vi "dfd_Lattice Level Down.vi"(0 "Bm(z)":dbl[](array[numeric]) format="%.2f") -> (1 "Bm-1(z)":dbl[](array[numeric]) format="%.2f", 2 "km":dbl format="%.2f", 3 "fail?":bool)   [LabVIEW 2017, in "NI_DigFilterLicensed.lvlib"]
uses:
  <vilib>/addons/Digital Filter Design/NI_DigFilterLicensed.lvlib
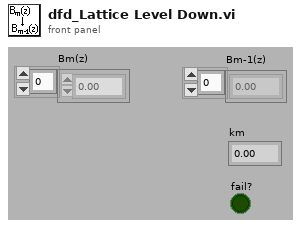
[diagram p1: front panel]
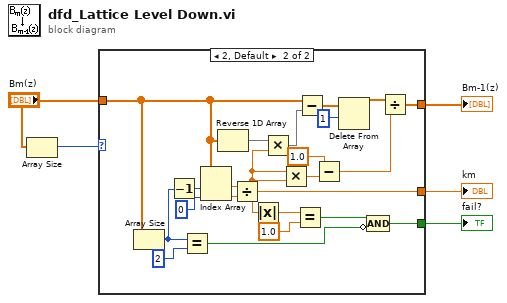
[diagram p0: block diagram]
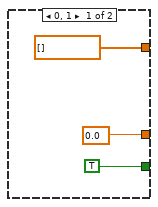
[diagram p2: hidden frame]
diagram:
  n1 = Array Size(array="Bm(z)") -> (size(s)=w1:i32)
  n2 = case shown="2, Default" w1 {
    tunnel: [TRUE w28] -> w5
    tunnel: "Bm(z)" -> [_ w27]
    tunnel: [dbl[] [] w9] -> w3
    tunnel: [0.0 ("Numeric") w10] -> w2
    frame 0, 1 {
    }
    frame 2, Default {
      n3 = Array Size(array=w27) -> (size(s)=w25:i32)
      n4 = Decrement(x=w25) -> (x-1=w24:i32)
      n5 = Equal?(x=w25, y=2) -> (x = y?=w29:bool)
      n6 = Index Array(array=w27, index #1=w24, index #2=0 ("index")) -> (element #1=w21:dbl, element #2=w22:dbl)
      n7 = Reverse 1D Array(array=w27) -> (reversed array=w16:dbl[])
      n8 = Divide(x=w21, y=w22) -> (x/y=w10:dbl)
      n9 = Absolute Value(x=w10) -> (abs(x)=w19:dbl)
      n10 = Multiply(x=w16, y=w10) -> (x*y=w15:dbl[])
      n11 = Multiply(x=w10, y=w10) -> (x*y=w18:dbl)
      n12 = Equal?(x=w19, y=1.0) -> (x = y?=w30:bool)
      n13 = Subtract(x=w27, y=w15) -> (x-y=w14:dbl[])
      n14 = Subtract(x=1.0, y=w18) -> (x-y=w13:dbl)
      n15 = Delete From Array(array=w14, length=1 ("index")) -> (array with subset deleted=w11:dbl[])  [unwired: 1 in, 1 out]
      n16 = Compound Arithmetic op=AND(w30, invert w29) -> (w28:bool)
      n17 = Divide(x=w11, y=w13) -> (x/y=w9:dbl[])
    }
  }
  "Bm-1(z)" <- w3
  "km" <- w2
  "fail?" <- w5
